vi "XY Graph Select Plots... Event.vi"(8 "Error In":errorcluster, 10 "Select (T)/Deselect":bool=TRUE, 11 "XYGraph Ref":T1) -> (0 "Error Out":errorcluster, 1 "Message":string, 2 "Plot Names":string[](array[string]), 3 "XYGraph Ref":T1, 5 "Graph Caption":string)   [LabVIEW 2019, in "XY Graph Add-Ons.lvlib"]
uses:
  XY Graph Add-Ons.lvlib
  XY Graph Refnum.ctl
  <vilib>/Utility/High Resolution Relative Seconds.vi
panel:
  out "CPU (s)":dbl
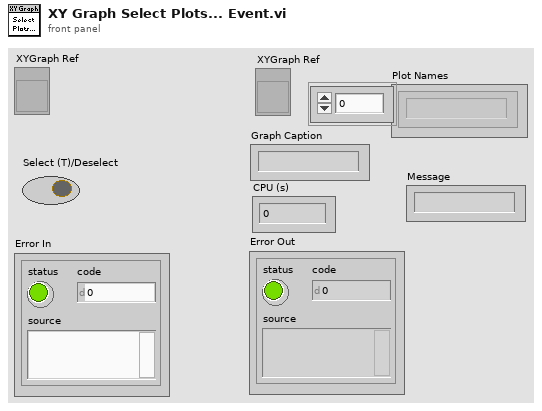
[diagram p1: front panel]
types:
  T1 = typedef "XY Graph Add-Ons.lvlib/XY Graph Refnum.ctl" = refnum<vi>
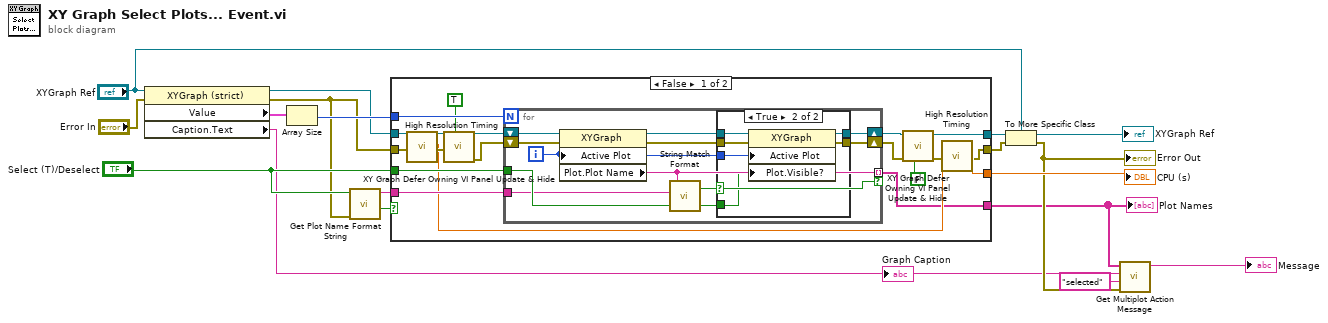
[diagram p0: block diagram]
diagram:
  n1 = property class="XYGraph (strict)"(reference="XYGraph Ref", error in="Error In") -> (reference out=w16:T1, error out=w7:errorcluster, "Value"=w18:cluster{"X Array":dbl[], "Y Array":dbl[]}[], "Caption.Text"=w4:string)
  "Graph Caption" <- w4
  n2 = Array Size(array=w18) -> (size(s)=w17:i32)
  n3 = call "Get Plot Name Format String.vi"("error in (no error)"=w7, "Select(T)/Deselect(F)"="Select (T)/Deselect") -> ("Cancelled?"=w8:bool, "String Format"=w10:string)  [unwired: 7 in, 1 out]
  n4 = case shown="False" w8 {
    tunnel: w17 -> [w36 _]
    tunnel: w16 -> [w35 w57]
    tunnel: [w30 w57] -> w14
    tunnel: [w21 w56] -> w11
    tunnel: w10 -> [w28 _]
    tunnel: "Select (T)/Deselect" -> [w27 _]
    tunnel: w7 -> [w24 w56]
    tunnel: [w22 _] -> w6
    tunnel: [w19 _] -> w2
    frame False {
      n5 = call "High Resolution Timing.vi"("Error In"=w24) -> ("elapsed (relative) seconds"=w20:dbl, "Error Out"=w23:errorcluster)  [unwired: 16 in, 1 out]
      n6 = call "XY Graph Defer Owning VI Panel Update & Hide.vi"("Defer Owning Panel Update"=TRUE ("Hide (F)/Show (T) Graph"), "error in (no error)"=w23, "XY Graph Refnum in"=w35) -> ("error out"=w33:errorcluster, "XY Graph Refnum out"=w34:refnum<vi>)  [unwired: 7 in]
      n7 = for {
        N: w36 -> [_]
        shift-right: [w47] -> w32
        shift-left: w34 -> [w44]
        shift-right: [w46] -> w31
        shift-left: w33 -> [w43]
        tunnel: w27 -> [w40]
        tunnel: w28 -> [w39]
        tunnel: [w38] -> w19 mode=indexing if=w37
        i -> [w45]
        n8 = property class="XYGraph"(reference=w44, error in=w43, "Active Plot"=w45) -> (reference out=w42:refnum<vi>, error out=w41:errorcluster, "Plot.Plot Name"=w38:string)
        n9 = call "String Match Format.vi"("String Format"=w39, "String"=w38) -> ("Match format?"=w37:bool)  [unwired: 3 in]
        n10 = case shown="True" w37 {
          tunnel: [w49 w55] -> w47
          tunnel: [w48 w54] -> w46
          tunnel: w45 -> [_ w53]
          tunnel: w42 -> [w49 w52]
          tunnel: w41 -> [w48 w51]
          tunnel: w40 -> [_ w50]
          frame False {
          }
          frame True {
            n11 = property class="XYGraph"(reference=w52, error in=w51, "Active Plot"=w53, "Plot.Visible?"=w50) -> (reference out=w55:refnum<vi>, error out=w54:errorcluster)
          }
        }
      }
      n12 = call "XY Graph Defer Owning VI Panel Update & Hide.vi"("Defer Owning Panel Update"=FALSE ("Hide (F)/Show (T) Graph"), "error in (no error)"=w31, "XY Graph Refnum in"=w32) -> ("error out"=w29:errorcluster, "XY Graph Refnum out"=w30:refnum<vi>)  [unwired: 7 in]
      n13 = call "High Resolution Timing.vi"("relative seconds (NaN)"=w20, "Error In"=w29) -> ("elapsed (relative) seconds"=w22:dbl, "Error Out"=w21:errorcluster)  [unwired: 15 in, 1 out]
    }
    frame True {
    }
  }
  "CPU (s)" <- w6
  "Plot Names" <- w2
  n14 = To More Specific Class(target class="XYGraph Ref", reference=w14, error in=w11) -> (specific class reference=→"XYGraph Ref":T1, error out=w5:errorcluster)
  "Error Out" <- w5
  n15 = call "Get Multiplot Action Message.vi"("error in (no error)"=w5, "Graph Action"="selected", "Graph Caption"=w4, "Plot Names"=w2) -> ("Multiplot Message"=→"Message":string)  [unwired: 6 in, 1 out]
